vi "Verify.vi"(5 "Options":T1, 7 "Test VI (caller)":string, 8 "error in":errorcluster, 10 "Test Data":string, 11 "LUnit Test Case In":refnum<class "Test Case.lvclass">) -> (0 "error out":errorcluster, 3 "LUnit Test Case Out":refnum<class "Test Case.lvclass">)   [LabVIEW 2020, in "LUnitExtension.lvlib"]
doc: "Takes in anything. With default printer, it needs to be a string or it will error out. With the correct printer, you can pass in anything, in that case you are responsible for providing the printer class that will decode the variant in and flatten to some reasonable string."
uses:
  LUnitExtension.lvlib
  <vilib>/Astemes/LUnit/Test Case.lvclass
  Approval Tests/Options.ctl
  Approval Tests/Reporter/Reporter.lvclass
  <vilib>/Astemes/LUnit/Test Case.lvclass/Test Case.ctl
  <vilib>/Astemes/LUnit/Append Fail Result.vi
  <vilib>/Astemes/LUnit/Append Pass Result.vi
  Approval Tests/Approval Tests.lvlib
  77738755-7f98-4f87-abc3-57aa04d1f56f.vi
  Approval Tests/Printer/Printer.lvclass
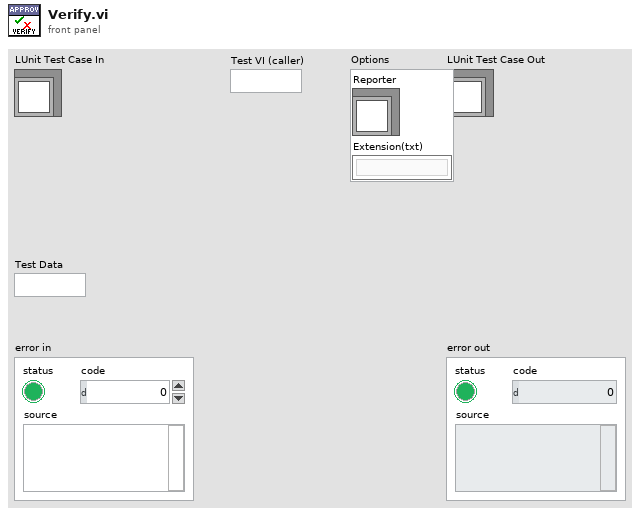
[diagram p1: front panel]
types:
  T1 = typedef "Approval Tests.lvlib/Options.ctl" = cluster{"Reporter":refnum<class "Reporter.lvclass">, "Extension(txt)":string}
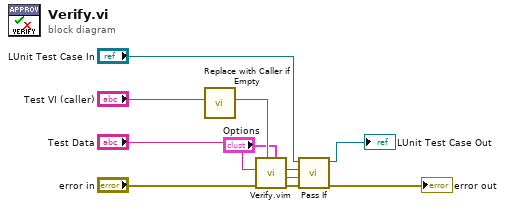
[diagram p0: block diagram]
diagram:
  n1 = call "Replace with Caller if Empty.vi"("Test VI (caller) in"="Test VI (caller)") -> ("Test VI (caller) out"=w2:string)  [unwired: 10 in]
  n2 = call "Verify.vim"("Options"="Options", "Test VI (caller)"=w2, "error in"="error in", "Anything"="Test Data") -> ("error out"=w9:errorcluster, "Failure Message"=w4:string, "Passed?"=w5:bool)  [unwired: 5 in]
  n3 = call <vilib>:"Pass If.vi"("error in (no error)"=w9, "Message"=w4, "Pass?"=w5, "LUnit Test Case In"="LUnit Test Case In") -> ("error out"=→"error out":errorcluster, "LUnit Test Case Out"=→"LUnit Test Case Out":refnum<class "Test Case.lvclass">)  [unwired: 6 in]
